vi "CustomDataHelperGraph.vi"(0 "object in":refnum<class "AD2_DO_SDK.lvclass">, 1 "ExitExternalPrograms":refnum<notifier>, 2 "Pulse Settings":T1={"Pulse Length(ms)"=7.0, "DIO0Offset(ms)"=1.0, "DIO1 Pulse time (ms)"=2.0, "DIO2 Pulse time (ms) 2"=30.0, "DIO3 Pulse time (ms) 3"=0.0, "EnableDIO3"=FALSE, "EnableDIO2"=TRUE, "EnableDIO1"=TRUE}, 3 "Exposure Time (ms)":dbl=4.0, 4 "ReadoutTime":dbl=1.0, 5 "error in (no error)":errorcluster) -> (14 "object out":refnum<class "AD2_DO_SDK.lvclass">, 19 "error out":errorcluster)   [LabVIEW 2021, in "AD2_DO_SDK.lvclass"]
doc: "This VI doest the same as DOconfigureCustomPattern but With a different Front panel. It is custom-made for the IAF Cytometer application"
uses:
  AD2_DO_SDK.lvclass
  DOConfigureCustomData.ctl
  DOTrigger.ctl
  AD2_WFG_SDK_class/AD2TriggerSources.ctl
  DOCustomData.ctl
  AD2_SDK_class/AD2_SDK.lvclass
panel:
  in  "Tab Control":enum32{"Helper", "Ilustration"}(tab)
  out "Waveform Graph":dbl[][](graph)=[[0.0, 0.0, 0.0, 1.0, 1.0, 1.0, 1.0, 1.0, 1.0, 1.0, 0.0, 0.0, 0.0, 0.0, 0.0, 0.0, 0.0, 0.0, 0.0, 0.0, 0.0, 0.0, 0.0, 0.0, 0.0, 0.0, 0.0, 0.0, 0.0, 0.0, 0.0, 1.0, 1.0, 1.0, 1.0, 1.0, 1.0, 1.0, 0.0, 0.0, 0.0, 0.0, 0.0, 0.0], [0.0, 0.0, 1.1, 1.1, 1.1, 1.1, 1.1, 1.1, 1.1, 0.0, 0.0, 0.0, 0.0, 0.0, 0.0, 0.0, 0.0, 0.0, 0.0, 0.0, 0.0, 0.0, 0.0, 0.0, 0.0, 0.0, 0.0, 0.0, 0.0, 0.0, 0.0, 0.0, 0.0, 0.0, 0.0, 0.0, 0.0, 0.0, 0.0, 0.0, 0.0, 0.0, 0.0, 0.0], [0.0, 0.0, 0.0, 0.0, 0.0, 0.0, 0.0, 0.0, 0.0, 0.0, 0.0, 0.0, 0.0, 0.0, 0.0, 0.0, 0.0, 0.0, 0.0, 0.0, 0.0, 0.0, 0.0, 0.0, 0.0, 0.0, 0.0, 0.0, 0.0, 0.0, 1.2, 1.2, 1.2, 1.2, 1.2, 1.2, 1.2, 0.0, 0.0, 0.0, 0.0, 0.0, 0.0, 0.0], [0.0, 0.0, 0.0, 0.0, 0.0, 0.0, 0.0, 0.0, 0.0, 0.0, 0.0, 0.0, 0.0, 0.0, 0.0, 0.0, 0.0, 0.0, 0.0, 0.0, 0.0, 0.0, 0.0, 0.0, 0.0, 0.0, 0.0, 0.0, 0.0, 0.0, 0.0, 0.0, 0.0, 0.0, 0.0, 0.0, 0.0, 0.0, 0.0, 0.0, 0.0, 0.0, 0.0, 0.0], [0.0, 0.0, 0.0, 1.4, 1.4, 1.4, 1.4, 0.0, 0.0, 0.0, 0.0, 0.0, 0.0, 0.0, 0.0, 0.0, 0.0, 0.0, 0.0, 0.0, 0.0, 0.0, 0.0, 0.0, 0.0, 0.0, 0.0, 0.0, 0.0, 0.0, 0.0, 1.4, 1.4, 1.4, 1.4, 0.0, 0.0, 0.0, 0.0, 0.0, 0.0, 0.0, 0.0, 0.0], [0.0, 0.0, 0.0, 0.0, 0.0, 0.0, 0.0, 1.5, 0.0, 0.0, 0.0, 0.0, 0.0, 0.0, 0.0, 0.0, 0.0, 0.0, 0.0, 0.0, 0.0, 0.0, 0.0, 0.0, 0.0, 0.0, 0.0, 0.0, 0.0, 0.0, 0.0, 0.0, 0.0, 0.0, 0.0, 1.5, 0.0, 0.0, 0.0, 0.0, 0.0, 0.0, 0.0, 0.0]]
  out "appended array":bool[][](array[boolean])=[[FALSE, FALSE, FALSE, TRUE, TRUE, TRUE, TRUE, TRUE, TRUE, TRUE, FALSE, FALSE, FALSE, FALSE, FALSE, FALSE, FALSE, FALSE, FALSE, FALSE, FALSE, FALSE, FALSE, FALSE, FALSE, FALSE, FALSE, FALSE, FALSE, FALSE, FALSE, TRUE, TRUE, TRUE, TRUE, TRUE, TRUE, TRUE, FALSE, FALSE, FALSE, FALSE, FALSE, FALSE], [FALSE, FALSE, TRUE, TRUE, TRUE, TRUE, TRUE, TRUE, TRUE, FALSE, FALSE, FALSE, FALSE, FALSE, FALSE, FALSE, FALSE, FALSE, FALSE, FALSE, FALSE, FALSE, FALSE, FALSE, FALSE, FALSE, FALSE, FALSE, FALSE, FALSE, FALSE, FALSE, FALSE, FALSE, FALSE, FALSE, FALSE, FALSE, FALSE, FALSE, FALSE, FALSE, FALSE, FALSE], [FALSE, FALSE, FALSE, FALSE, FALSE, FALSE, FALSE, FALSE, FALSE, FALSE, FALSE, FALSE, FALSE, FALSE, FALSE, FALSE, FALSE, FALSE, FALSE, FALSE, FALSE, FALSE, FALSE, FALSE, FALSE, FALSE, FALSE, FALSE, FALSE, FALSE, TRUE, TRUE, TRUE, TRUE, TRUE, TRUE, TRUE, FALSE, FALSE, FALSE, FALSE, FALSE, FALSE, FALSE], [FALSE, FALSE, FALSE, FALSE, FALSE, FALSE, FALSE, FALSE, FALSE, FALSE, FALSE, FALSE, FALSE, FALSE, FALSE, FALSE, FALSE, FALSE, FALSE, FALSE, FALSE, FALSE, FALSE, FALSE, FALSE, FALSE, FALSE, FALSE, FALSE, FALSE, FALSE, FALSE, FALSE, FALSE, FALSE, FALSE, FALSE, FALSE, FALSE, FALSE, FALSE, FALSE, FALSE, FALSE], [FALSE, FALSE, FALSE, TRUE, TRUE, TRUE, TRUE, FALSE, FALSE, FALSE, FALSE, FALSE, FALSE, FALSE, FALSE, FALSE, FALSE, FALSE, FALSE, FALSE, FALSE, FALSE, FALSE, FALSE, FALSE, FALSE, FALSE, FALSE, FALSE, FALSE, FALSE, TRUE, TRUE, TRUE, TRUE, FALSE, FALSE, FALSE, FALSE, FALSE, FALSE, FALSE, FALSE, FALSE], [FALSE, FALSE, FALSE, FALSE, FALSE, FALSE, FALSE, TRUE, FALSE, FALSE, FALSE, FALSE, FALSE, FALSE, FALSE, FALSE, FALSE, FALSE, FALSE, FALSE, FALSE, FALSE, FALSE, FALSE, FALSE, FALSE, FALSE, FALSE, FALSE, FALSE, FALSE, FALSE, FALSE, FALSE, FALSE, TRUE, FALSE, FALSE, FALSE, FALSE, FALSE, FALSE, FALSE, FALSE]]
  in  "Exit Pulse Helper":bool
  # "DIO0 Pulses at the same time as DIO1,2 and 3 +-offset\nSet Pulse Length > exposure time+readout time"
  # "DIO0 (camera)"
  # "DIO1 (COOL-LED CH1)"
  # "DIO2 (COOL-LED CH2)"
  # "DIO3 (COOL-LED CH3)"
  # "Each Element is 1ms"
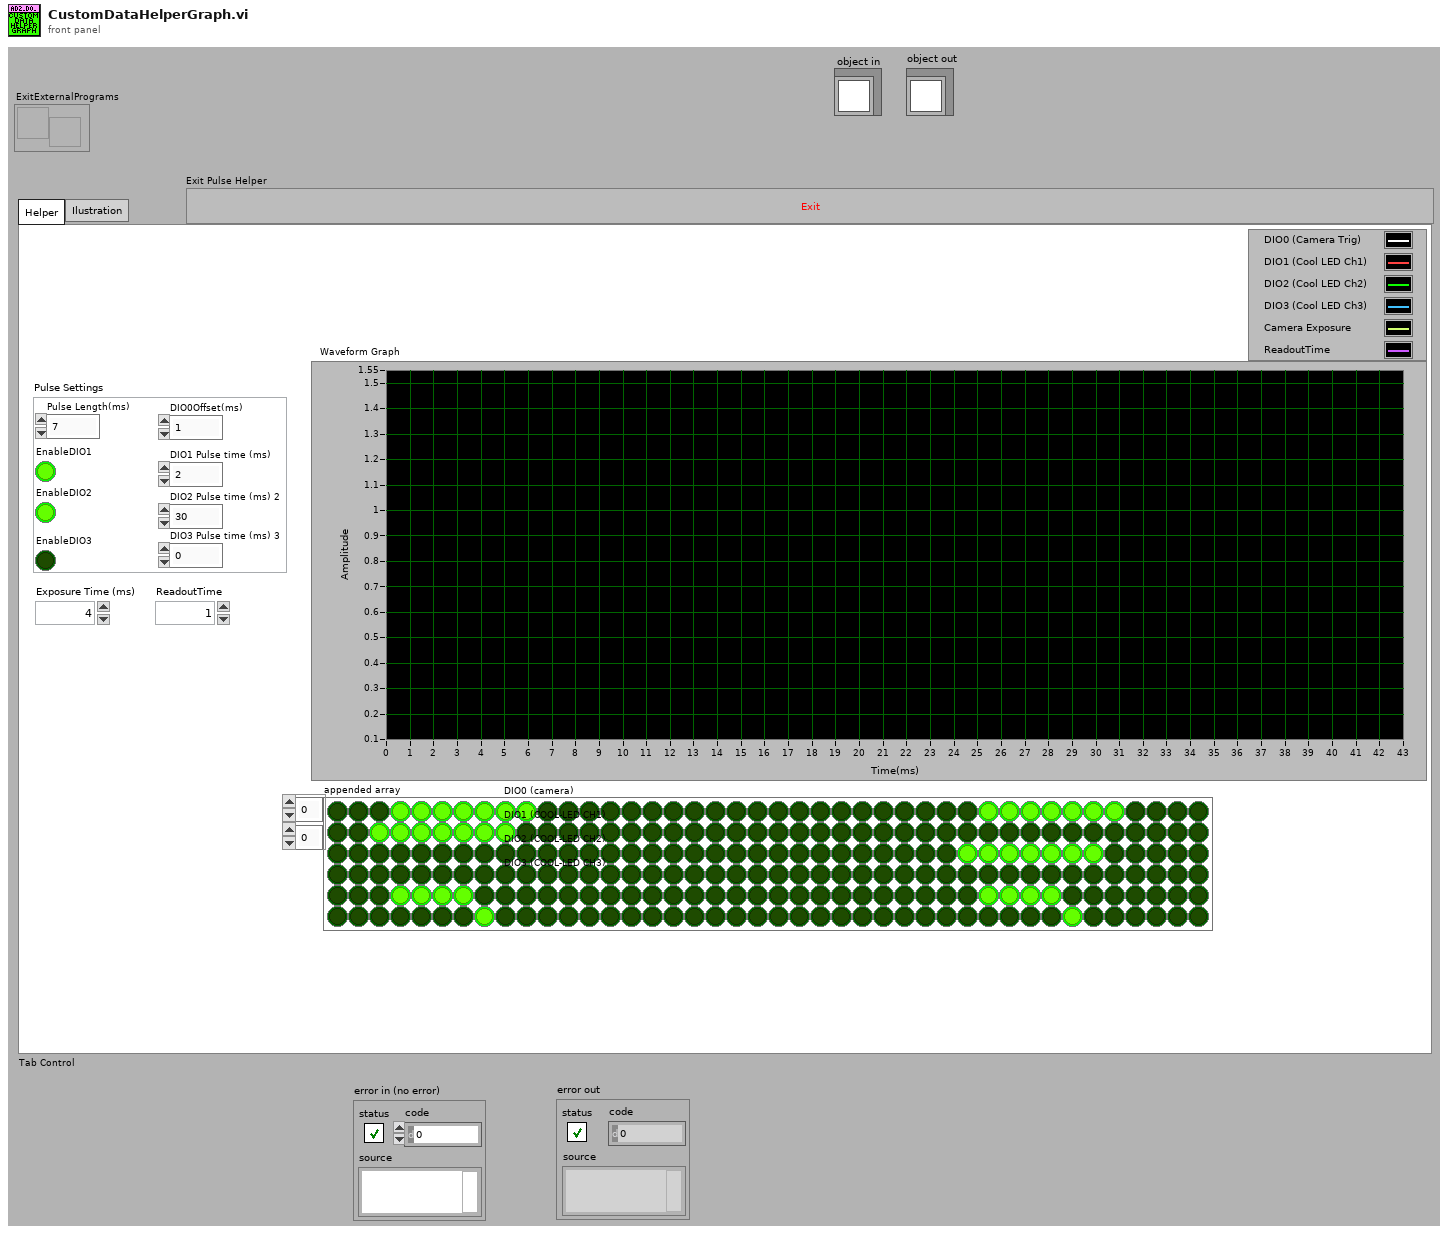
[diagram p1: front panel]
types:
  T1 = cluster{"Pulse Length(ms)":dbl, "DIO0Offset(ms)":dbl, "DIO1 Pulse time (ms)":dbl, "DIO2 Pulse time (ms) 2":dbl, "DIO3 Pulse time (ms) 3":dbl, "EnableDIO3":bool, "EnableDIO2":bool, "EnableDIO1":bool}
  T2 = typedef "AD2_SDK.lvclass/AD2TriggerSources.ctl" = enum8{"trigrsrcNone", "trigsrcPC", "trigsrcDetectorAnalogIn", "trigsrcDetectorDigitalIn", "trigsrcAnalogIn", "trigsrcDigitalIn", "trigsrcDigitalOut", "trigsrcAnalogOut1", "trigsrcAnalogOut2", "trigsrcAnalogOut3", "trigsrcAnalogOut4", "trigsrcExternal1", "trigsrcExternal2", "trigsrcExternal3", "trigsrcExternal4", ""}
  T3 = typedef "AD2_DO_SDK.lvclass/DOCustomData.ctl" = cluster{"Data":bool[], "Freq":dbl, "#Bits":u32, "Enable":bool, "IdleState":u16}[]
  T4 = typedef "AD2_DO_SDK.lvclass/DOTrigger.ctl" = cluster{"secRun(0=Cont)":dbl, "secWait":dbl, "cRepeat(0=inf)":i32, "Repeat Trigger":bool, "TrigrSrc":T2}
  T5 = typedef "DOConfigureCustomData.ctl" = cluster{"DO Trigger":T4, "CustomData":T3}
  T6 = cluster{"Data":bool[], "Freq":dbl, "#Bits":u32, "Enable":bool, "IdleState":u16}
  T7 = cluster{"Data":bool[], "Freq":dbl, "#Bits":u32, "Enable":bool, "IdleState":u16}[]
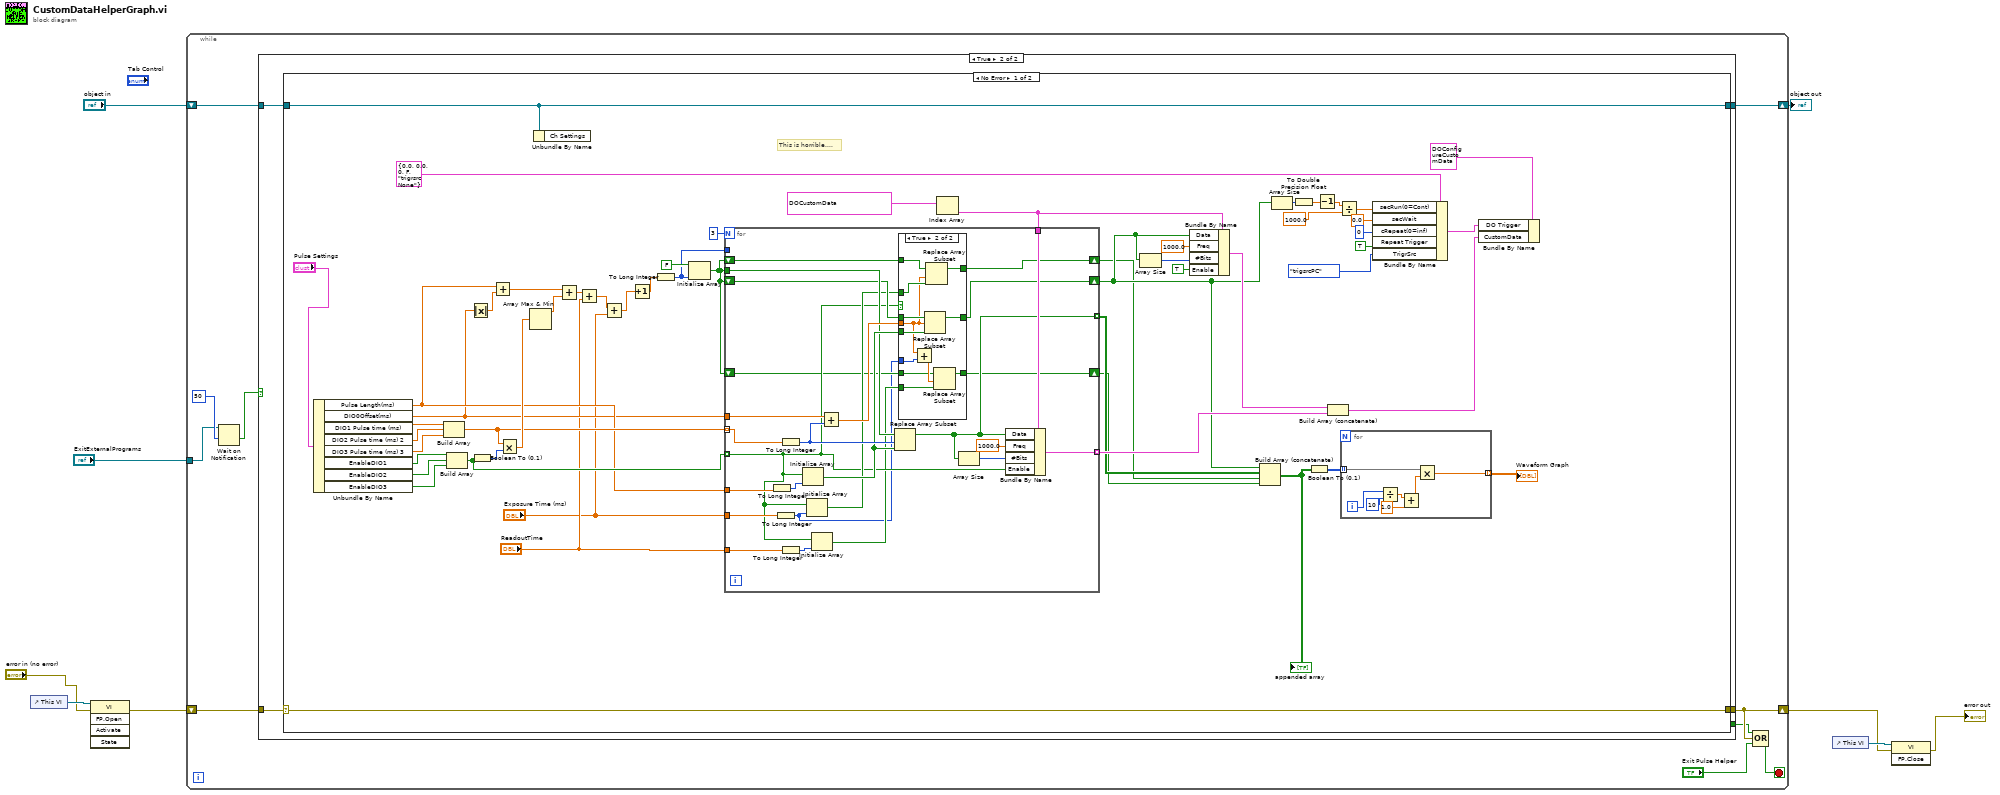
[diagram p0: block diagram]
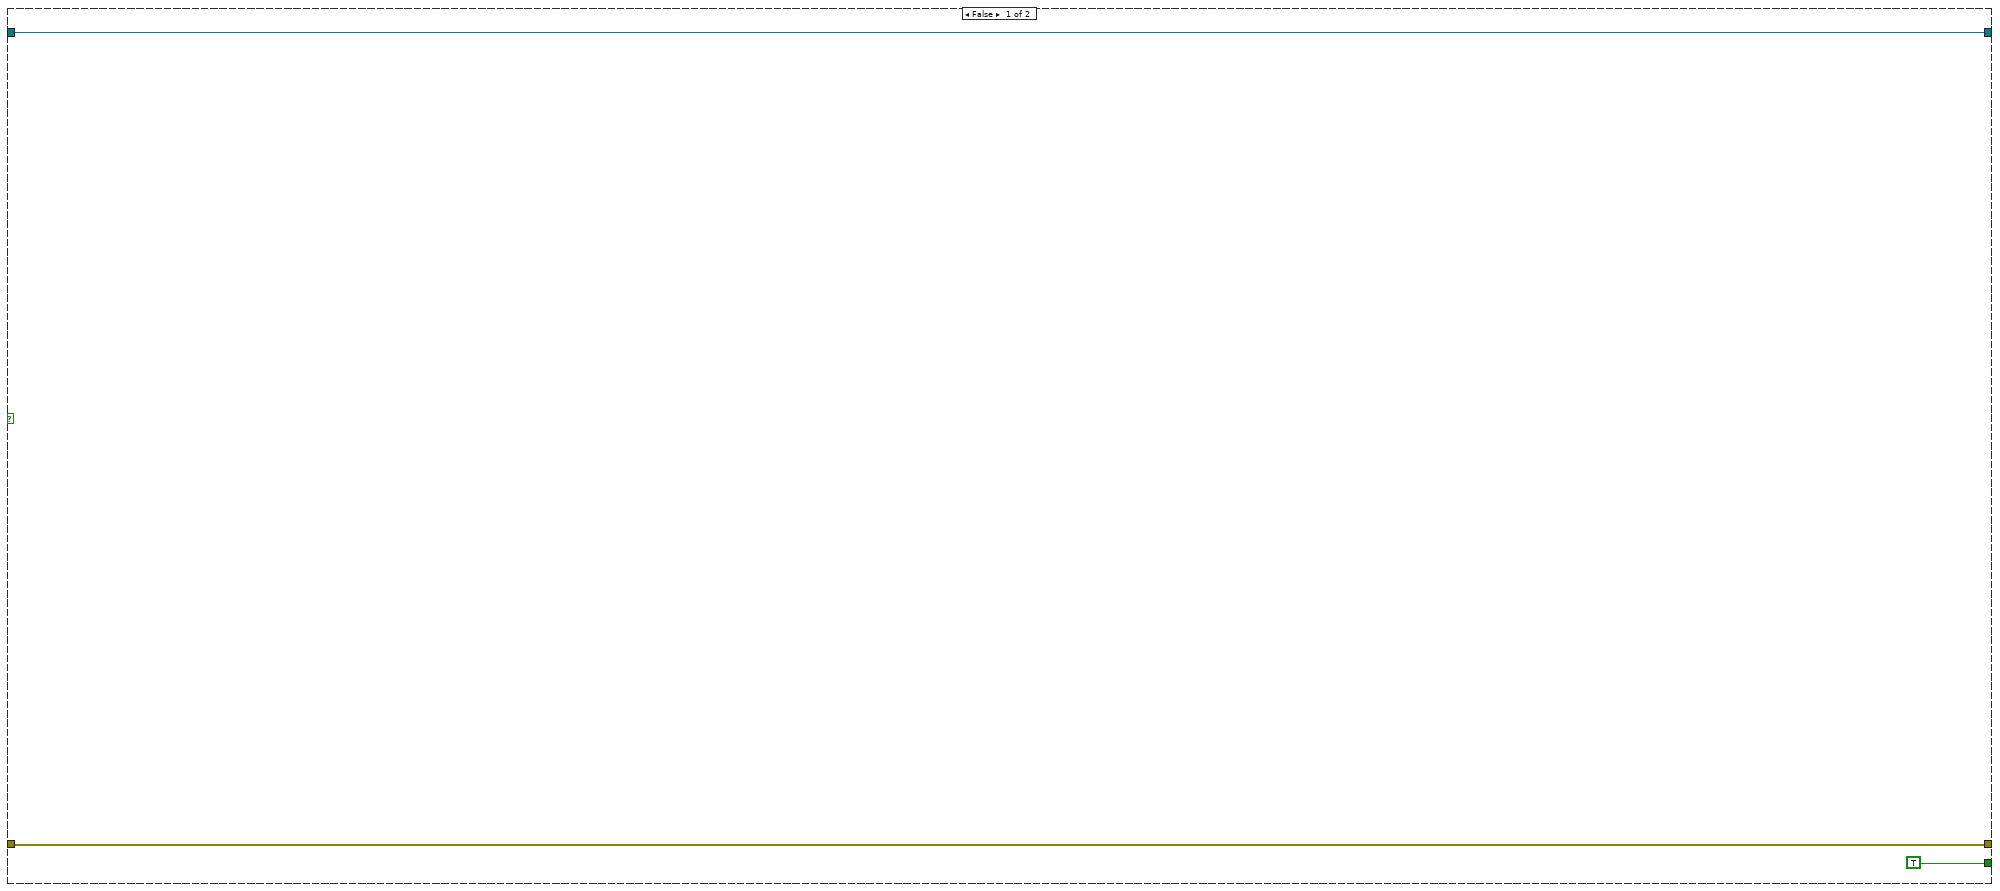
[diagram p2: hidden frame]
diagram:
  n1 = control-ref of="This VI"() -> (w4:refnum<vi>)
  n2 = invoke class="VI" method="FP.Open"(reference=w4, error in="error in (no error)") -> (error out=w2:errorcluster)  [unwired: 3 in, 4 out]
  n3 = while {
    shift-right: [w11] -> w6
    shift-left: w2 -> [w19]
    shift-right: [w17] -> w8
    shift-left: "object in" -> [w18]
    tunnel: "ExitExternalPrograms" -> [w15]
    stop <- w12 stop-if-true
    n4 = Wait on Notification(notifier=w15, timeout in ms (-1)=u32 50 ("millisecond multiple")) -> (timed out?=w14:bool)  [unwired: 2 in, 3 out]
    n5 = case shown="True" w14 {
      tunnel: w19 -> [w21 w26]
      tunnel: [w21 w25] -> w11
      tunnel: w18 -> [w22 w24]
      tunnel: [w22 w23] -> w17
      tunnel: [TRUE _] -> w10
      frame False {
      }
      frame True {
        n6 = case shown="No Error" w26 {
          selector: w26 -> [w41 w131]
          tunnel: [w41 w131] -> w25
          tunnel: [w42 w130] -> w23
          tunnel: w24 -> [w42 w130]
          frame No Error {
            # "This is horrible...."
            n7 = Unbundle By Name("Pulse Settings") -> ("Pulse Length(ms)"=w63:dbl, "DIO0Offset(ms)"=w61:dbl, "DIO1 Pulse time (ms)"=w64:dbl, "DIO2 Pulse time (ms) 2"=w73:dbl, "DIO3 Pulse time (ms) 3"=w72:dbl, "EnableDIO1"=w76:bool, "EnableDIO2"=w75:bool, "EnableDIO3"=w74:bool)
            n8 = Build Array(w64, w73, w72) -> (w67:dbl[])
            n9 = Build Array(w76, w75, w74) -> (w66:bool[])
            n10 = Absolute Value(x=w61) -> (abs(x)=w60:dbl)
            n11 = Boolean To (0,1)(Boolean=w66) -> (0, 1=w71:i16[])
            n12 = Add(x=w63, y=w60) -> (x+y=w62:dbl)
            n13 = Multiply(x=w67, y=w71) -> (x*y=w70:dbl[])
            n14 = Array Max & Min(array=w70) -> (max value=w69:dbl)  [unwired: 3 out]
            n15 = Unbundle By Name(w42) -> ()  [unwired: 1 out]
            n16 = Add(x=w62, y=w69) -> (x+y=w30:dbl)
            n17 = Add(x=w30, y="ReadoutTime") -> (x+y=w29:dbl)
            n18 = Add(x=w29, y="Exposure Time (ms)") -> (x+y=w28:dbl)
            n19 = Increment(x=w28) -> (x+1=w44:dbl)
            n20 = To Long Integer(number=w44) -> (32bit integer=w56:i32)
            n21 = Initialize Array(FALSE, w56) -> (w33:bool[])
            n22 = Index Array(array=T3 [{"Data"=[], "Freq"=0.0, "#Bits"=0, "Enable"=FALSE, "IdleState"=0}, {"Data"=[], "Freq"=0.0, "#Bits"=0, "Enable"=FALSE, "IdleState"=0}, {"Data"=[], "Freq"=0.0, "#Bits"=0, "Enable"=FALSE, "IdleState"=0}, {"Data"=[FALSE, FALSE, FALSE, FALSE, FALSE, FALSE, FALSE, FALSE, FALSE, FALSE, FALSE, FALSE, FALSE, FALSE, FALSE, FALSE, FALSE, FALSE, FALSE, FALSE, FALSE, FALSE, FALSE], "Freq"=0.0, "#Bits"=0, "Enable"=FALSE, "IdleState"=0}, {"Data"=[], "Freq"=0.0, "#Bits"=0, "Enable"=FALSE, "IdleState"=0}, {"Data"=[], "Freq"=0.0, "#Bits"=0, "Enable"=FALSE, "IdleState"=0}, {"Data"=[], "Freq"=0.0, "#Bits"=0, "Enable"=FALSE, "IdleState"=0}, {"Data"=[], "Freq"=0.0, "#Bits"=0, "Enable"=FALSE, "IdleState"=0}, {"Data"=[], "Freq"=0.0, "#Bits"=0, "Enable"=FALSE, "IdleState"=0}, {"Data"=[], "Freq"=0.0, "#Bits"=0, "Enable"=FALSE, "IdleState"=0}, {"Data"=[], "Freq"=0.0, "#Bits"=0, "Enable"=FALSE, "IdleState"=0}, {"Data"=[], "Freq"=0.0, "#Bits"=0, "Enable"=FALSE, "IdleState"=0}, {"Data"=[], "Freq"=0.0, "#Bits"=0, "Enable"=FALSE, "IdleState"=0}, {"Data"=[], "Freq"=0.0, "#Bits"=0, "Enable"=FALSE, "IdleState"=0}, {"Data"=[], "Freq"=0.0, "#Bits"=0, "Enable"=FALSE, "IdleState"=0}, {"Data"=[FALSE, FALSE, FALSE, FALSE, FALSE, FALSE, FALSE, FALSE, FALSE, FALSE, FALSE, FALSE, FALSE, FALSE, FALSE, FALSE, FALSE, FALSE, FALSE, FALSE, FALSE, FALSE, FALSE], "Freq"=0.0, "#Bits"=0, "Enable"=FALSE, "IdleState"=0}, {"Data"=[FALSE, FALSE, FALSE, FALSE, FALSE, FALSE, FALSE, FALSE, FALSE, FALSE, FALSE, FALSE, FALSE, FALSE, FALSE, FALSE, FALSE, FALSE, FALSE, FALSE, FALSE, FALSE, FALSE], "Freq"=0.0, "#Bits"=0, "Enable"=FALSE, "IdleState"=0}] ("CustomData")) -> (element=w55:T6)  [unwired: 1 in]
            n23 = for {
              N: 3 -> [_]
              tunnel: w55 -> [w106]
              tunnel: w67 -> [w100] mode=indexing
              tunnel: w66 -> [w95] mode=indexing
              tunnel: w63 -> [w114]
              tunnel: w33 -> [w108]
              shift-right: [w105] -> w40
              shift-left: w33 -> [w107]
              tunnel: w61 -> [w111]
              tunnel: w56 -> [_]
              tunnel: [w103] -> w50 mode=indexing
              tunnel: [w101] -> w39 mode=indexing
              tunnel: "Exposure Time (ms)" -> [w99]
              shift-right: [w97] -> w34
              shift-left: w33 -> [w96]
              tunnel: "ReadoutTime" -> [w94]
              shift-right: [w91] -> w32
              shift-left: w33 -> [w92]
              n24 = To Long Integer(number=w114) -> (32bit integer=w113:i32)
              n25 = To Long Integer(number=w99) -> (32bit integer=w90:i32)
              n26 = To Long Integer(number=w100) -> (32bit integer=w112:i32)
              n27 = To Long Integer(number=w94) -> (32bit integer=w89:i32)
              n28 = Initialize Array(w95, w113) -> (w109:bool[])
              n29 = Initialize Array(w95, w90) -> (w98:bool[])
              n30 = Initialize Array(w95, w89) -> (w93:bool[])
              n31 = Add(x=w111, y=w112) -> (x+y=w110:dbl)
              n32 = Replace Array Subset(array=w108, new element=w109, index=w112) -> (w101:bool[])
              n33 = case shown="True" w95 {
                tunnel: w110 -> [_ w123]
                tunnel: w109 -> [_ w129]
                tunnel: w107 -> [w117 w127]
                tunnel: [w117 w128] -> w105
                tunnel: w98 -> [_ w126]
                tunnel: [w116 w125] -> w97
                tunnel: w96 -> [w116 w124]
                tunnel: w90 -> [_ w122]
                tunnel: w93 -> [_ w120]
                tunnel: w92 -> [w115 w119]
                tunnel: [w115 w118] -> w91
                frame False {
                }
                frame True {
                  n34 = Add(x=w123, y=w122) -> (x+y=w121:dbl)
                  n35 = Replace Array Subset(array=w127, new element=w129, index=w123) -> (w128:bool[])
                  n36 = Replace Array Subset(array=w124, new element=w126, index=w123) -> (w125:bool[])
                  n37 = Replace Array Subset(array=w119, new element=w120, index=w121) -> (w118:bool[])
                }
              }
              n38 = Array Size(array=w101) -> (size(s)=w102:i32)
              n39 = Bundle By Name(cluster=w106, "Data"=w101, "Freq"=1000.0, "#Bits"=w102, "Enable"=w95) -> (w103:T6)
            }
            n40 = Array Size(array=w40) -> (size(s)=w53:i32)
            n41 = Bundle By Name(cluster=w55, "Data"=w40, "Freq"=1000.0, "#Bits"=w53, "Enable"=TRUE) -> (w51:T6)
            n42 = Build Array (concatenate)(w40, w39, w34, w32) -> (w38:bool[][])
            "appended array" <- w38
            n43 = Array Size(array=w40) -> (size(s)=w57:i32)
            n44 = To Double Precision Float(number=w57) -> (double precision float=w46:dbl)
            n45 = Boolean To (0,1)(Boolean=w38) -> (0, 1=w37:i16[][])
            n46 = Decrement(x=w46) -> (x-1=w45:dbl)
            n47 = Build Array (concatenate)(w51, w50) -> (w49:T7)
            n48 = Divide(x=w45, y=1000.0) -> (x/y=w58:dbl)
            n49 = for {
              tunnel: w37 -> [w87] mode=indexing
              tunnel: [w86] -> w36 mode=indexing
              i -> [w85]
              n50 = Divide(x=w85, y=10) -> (x/y=w84:dbl)
              n51 = Add(x=w84, y=1.0) -> (x+y=w83:dbl)
              n52 = Multiply(x=w87, y=w83) -> (x*y=w86:dbl[])
            }
            "Waveform Graph" <- w36
            n53 = Bundle By Name(cluster=T4 {"secRun(0=Cont)"=0.0, "secWait"=0.0, "cRepeat(0=inf)"=0, "Repeat Trigger"=FALSE, "TrigrSrc"=enum."trigrsrcNone"} ("DO Trigger"), "secRun(0=Cont)"=w58, "secWait"=0.0, "cRepeat(0=inf)"=0, "Repeat Trigger"=TRUE, "TrigrSrc"=AD2TriggerSources."trigsrcPC") -> (w80:T4)
            n54 = Bundle By Name(cluster=T5 {"DO Trigger"={"secRun(0=Cont)"=0.1, "secWait"=0.0, "cRepeat(0=inf)"=0, "Repeat Trigger"=TRUE, "TrigrSrc"=enum."trigsrcPC"}, "CustomData"=[{"Data"=[FALSE, TRUE, FALSE, FALSE, FALSE, FALSE, FALSE, FALSE, FALSE, FALSE, FALSE, FALSE, TRUE, FALSE, FALSE, FALSE, FALSE, FALSE, FALSE, FALSE, FALSE, FALSE], "Freq"=1000.0, "#Bits"=1000, "Enable"=TRUE, "IdleState"=0}, {"Data"=[FALSE, FALSE, FALSE, FALSE, FALSE, FALSE, FALSE, FALSE, FALSE, FALSE, FALSE, FALSE, FALSE, FALSE, FALSE, FALSE, FALSE, FALSE, FALSE, FALSE, FALSE, FALSE], "Freq"=1000.0, "#Bits"=100, "Enable"=FALSE, "IdleState"=0}, {"Data"=[FALSE], "Freq"=0.0, "#Bits"=0, "Enable"=FALSE, "IdleState"=0}, {"Data"=[FALSE, FALSE, FALSE, FALSE, FALSE, FALSE, FALSE, FALSE, FALSE, FALSE, FALSE, FALSE, FALSE, FALSE, FALSE, FALSE, FALSE, FALSE, FALSE, FALSE, FALSE, FALSE, FALSE], "Freq"=0.0, "#Bits"=0, "Enable"=FALSE, "IdleState"=0}, {"Data"=[], "Freq"=0.0, "#Bits"=0, "Enable"=FALSE, "IdleState"=0}, {"Data"=[], "Freq"=0.0, "#Bits"=0, "Enable"=FALSE, "IdleState"=0}, {"Data"=[], "Freq"=0.0, "#Bits"=0, "Enable"=FALSE, "IdleState"=0}, {"Data"=[], "Freq"=0.0, "#Bits"=0, "Enable"=FALSE, "IdleState"=0}, {"Data"=[], "Freq"=0.0, "#Bits"=0, "Enable"=FALSE, "IdleState"=0}, {"Data"=[], "Freq"=0.0, "#Bits"=0, "Enable"=FALSE, "IdleState"=0}, {"Data"=[], "Freq"=0.0, "#Bits"=0, "Enable"=FALSE, "IdleState"=0}, {"Data"=[], "Freq"=0.0, "#Bits"=0, "Enable"=FALSE, "IdleState"=0}, {"Data"=[], "Freq"=0.0, "#Bits"=0, "Enable"=FALSE, "IdleState"=0}, {"Data"=[], "Freq"=0.0, "#Bits"=0, "Enable"=FALSE, "IdleState"=0}, {"Data"=[], "Freq"=0.0, "#Bits"=0, "Enable"=FALSE, "IdleState"=0}, {"Data"=[FALSE, FALSE, FALSE, FALSE, FALSE, FALSE, FALSE, FALSE, FALSE, FALSE, FALSE, FALSE, FALSE, FALSE, FALSE, FALSE, FALSE, FALSE, FALSE, FALSE, FALSE, FALSE, FALSE], "Freq"=0.0, "#Bits"=0, "Enable"=FALSE, "IdleState"=0}, {"Data"=[FALSE, FALSE, FALSE, FALSE, FALSE, FALSE, FALSE, FALSE, FALSE, FALSE, FALSE, FALSE, FALSE, FALSE, FALSE, FALSE, FALSE, FALSE, FALSE, FALSE, FALSE, FALSE, FALSE], "Freq"=0.0, "#Bits"=0, "Enable"=FALSE, "IdleState"=0}]}, "DO Trigger"=w80, "CustomData"=w49) -> ()  [unwired: 1 out]
          }
          frame Error {
          }
        }
      }
    }
    n55 = Compound Arithmetic op=OR(w10, w11, "Exit Pulse Helper") -> (w12:bool)
  }
  "object out" <- w8
  n56 = control-ref of="This VI"() -> (w7:refnum<vi>)
  n57 = invoke class="VI" method="FP.Close"(reference=w7, error in=w6) -> (error out=→"error out":errorcluster)  [unwired: 1 in, 2 out]
